vi "ДЗ.vi"   [LabVIEW 2021]
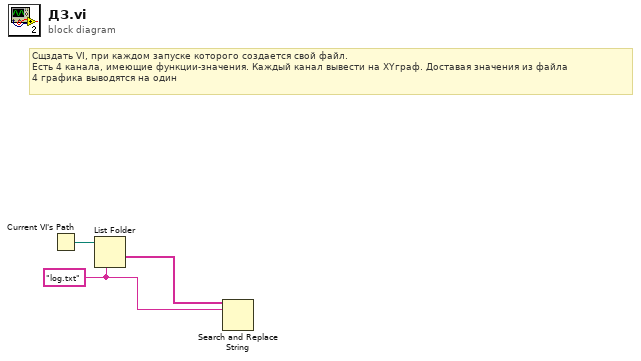
[diagram p0: block diagram]
diagram:
  w1 = "log.txt" ("pattern")
  # "Сщздать VI, при каждом запуске которого создается свой файл.\nЕсть 4 канала, имеющие функции-значения. Каждый канал вывести на XYграф. Доставая значения из файла\n4 графика выводятся на один"
  n1 = Current VI's Path() -> (path=w3:path)
  n2 = List Folder(path=w3, pattern=w1) -> (folder names=w2:string[])  [unwired: 2 in, 3 out]
  n3 = Search and Replace String(input string=w2, search string=w1) -> ()  [unwired: 6 in, 4 out]
